vi "20-tcoupl_type_bis.vi"(3 "this":i32, 4 "type in":i32, 5 "button":i32, 6 "settings in":T1={"Auto1"=TRUE, "Auto2"=TRUE, "Rel1"=TRUE, "Rel2"=TRUE, "Filt1"=TRUE, "Filt2"=TRUE, "Rate"=enum."Slow", "Range1"=enum."10mV", "Range2"=enum."100mV", "Filt3"=TRUE, "Filt4"=TRUE, "Rel temp 1"=TRUE, "Analog1"=FALSE, "Analog2"=FALSE, "Analog temp 1"=FALSE, "Digital1"=TRUE, "Digital2"=TRUE, "Digital temp 1 "=TRUE, "Window1"=enum."0,01%", "Window2"=enum."0,01%", "Window temp 1"=enum."0,01%", "RDGS1"="010", "RDGS2"="010", "RDGS temp 1"="010", "Type_type1"=TRUE, "Type_type2"=TRUE, "Type_type temp 1"=TRUE, "LSync"=FALSE, "Unit"=enum."C", "Sens"=TRUE, "Type tcoupl"=enum."J", "Junc"=TRUE, "prevState"=0, "Rel temp 2"=TRUE, "Analog temp 2"=FALSE, "Digital temp 2"=TRUE, "Type_type temp 2"=TRUE, "RDGS temp 2"="010", "Window temp 2"=enum."0,01%", "addres"=""}) -> (0 "next state":i32, 1 "type  out":i32, 2 "settings out":T1)   [LabVIEW 2017]
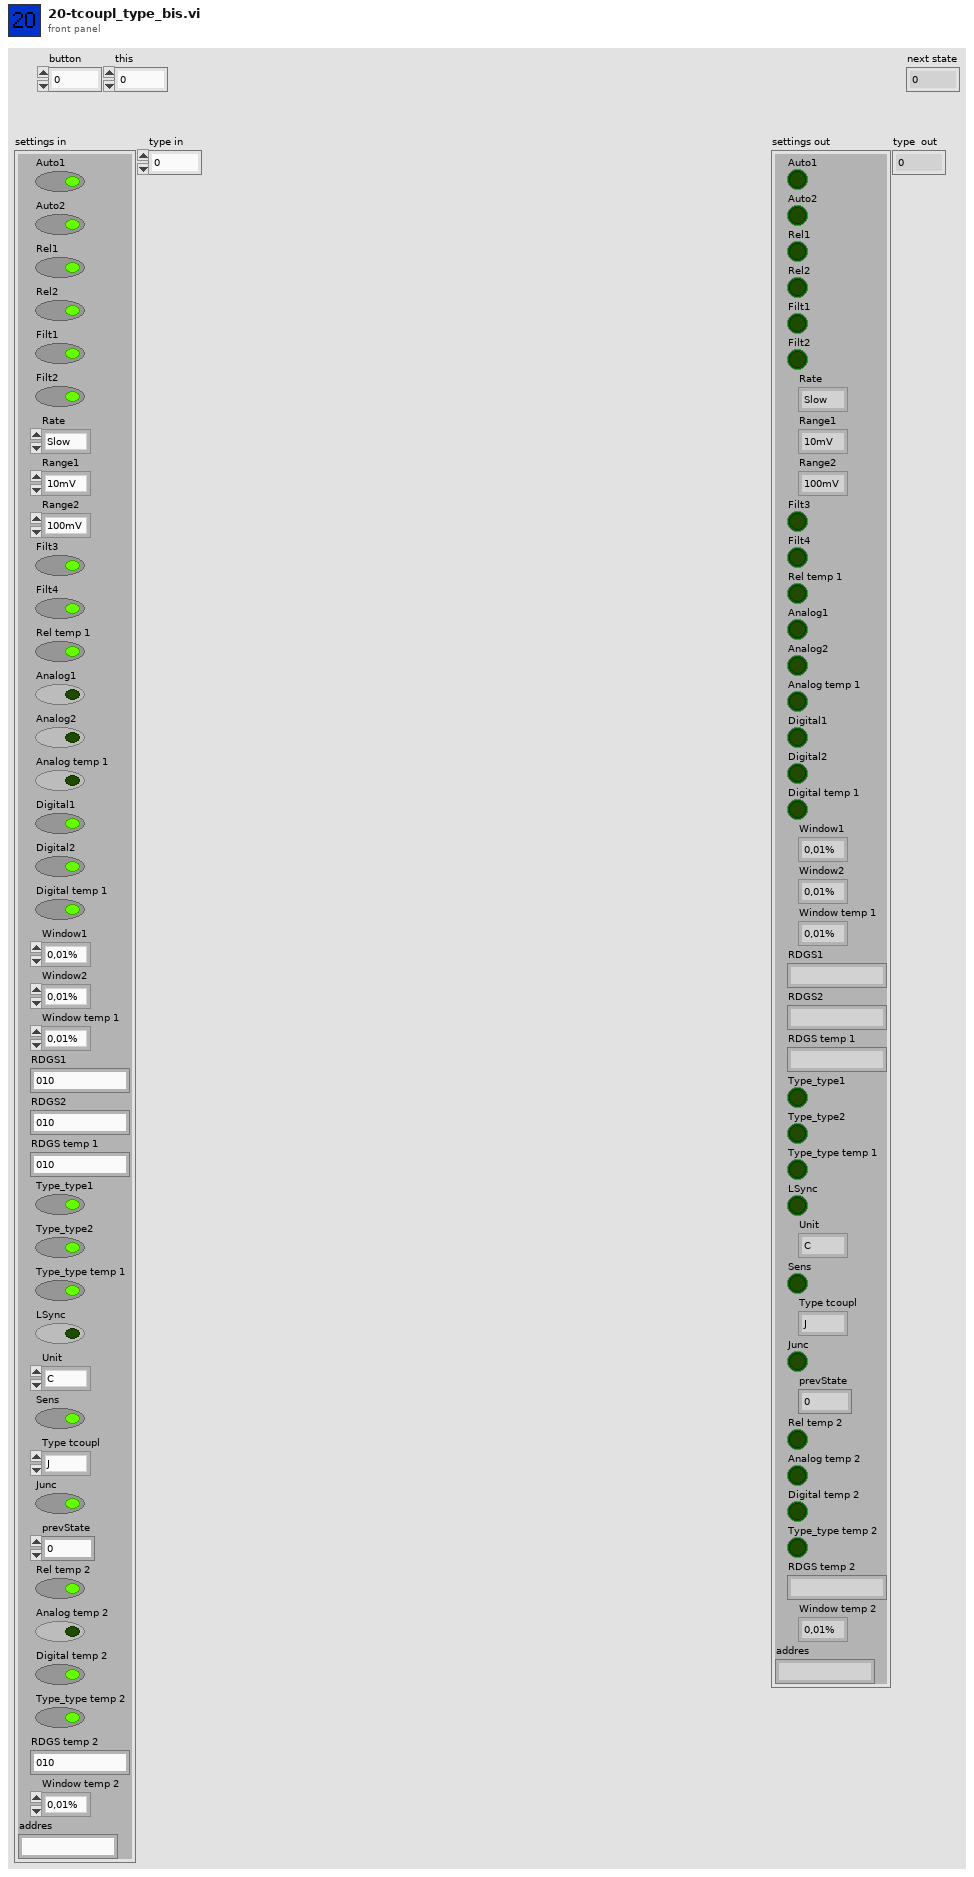
[diagram p1: front panel]
types:
  T1 = cluster{"Auto1":bool, "Auto2":bool, "Rel1":bool, "Rel2":bool, "Filt1":bool, "Filt2":bool, "Rate":enum16{"Slow", "Med", "Fast"}, "Range1":enum16{"10mV", "100mV", "1V", "10V", "100V"}, "Range2":enum16{"100mV", "1V", "10V"}, "Filt3":bool, "Filt4":bool, "Rel temp 1":bool, "Analog1":bool, "Analog2":bool, "Analog temp 1":bool, "Digital1":bool, "Digital2":bool, "Digital temp 1 ":bool, "Window1":enum16{"0,01%", "0,1%", "1%", "10%", "None"}, "Window2":enum16{"0,01%", "0,1%", "1%", "10%", "None"}, "Window temp 1":enum16{"0,01%", "0,1%", "1%", "10%", "None"}, "RDGS1":string, "RDGS2":string, "RDGS temp 1":string, "Type_type1":bool, "Type_type2":bool, "Type_type temp 1":bool, "LSync":bool, "Unit":enum16{"C", "K", "F"}, "Sens":bool, "Type tcoupl":enum16{"J", "K", "T", "E", "R", "S", "B", "N"}, "Junc":bool, "prevState":i32, "Rel temp 2":bool, "Analog temp 2":bool, "Digital temp 2":bool, "Type_type temp 2":bool, "RDGS temp 2":string, "Window temp 2":enum16{"0,01%", "0,1%", "1%", "10%", "None"}, "addres":string}
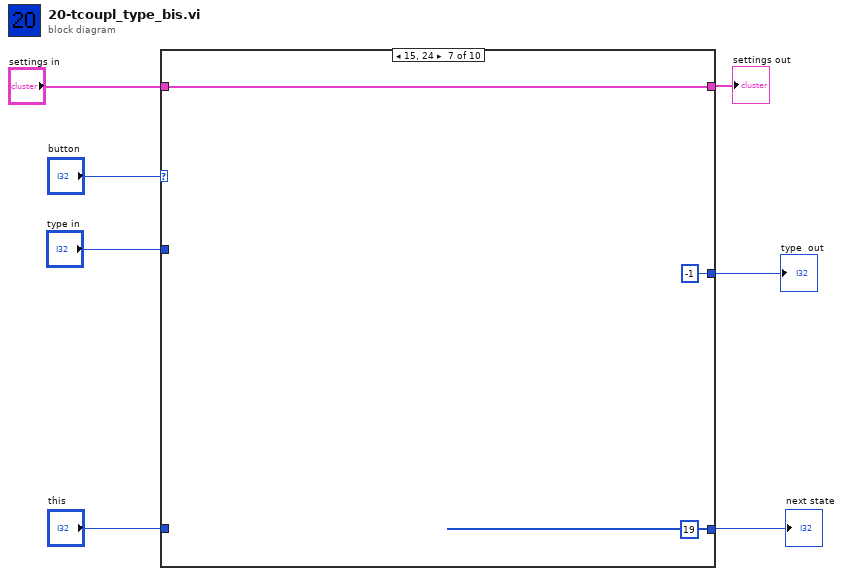
[diagram p0: block diagram]
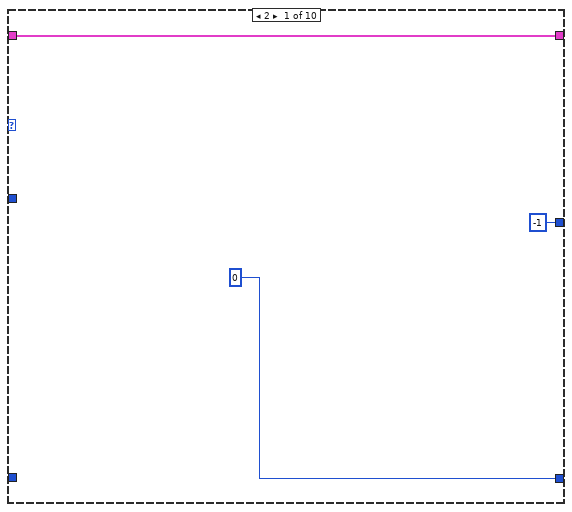
[diagram p2: hidden frame]
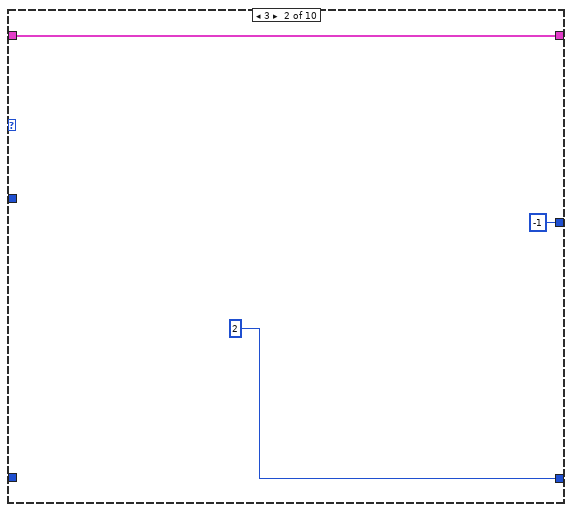
[diagram p3: hidden frame]
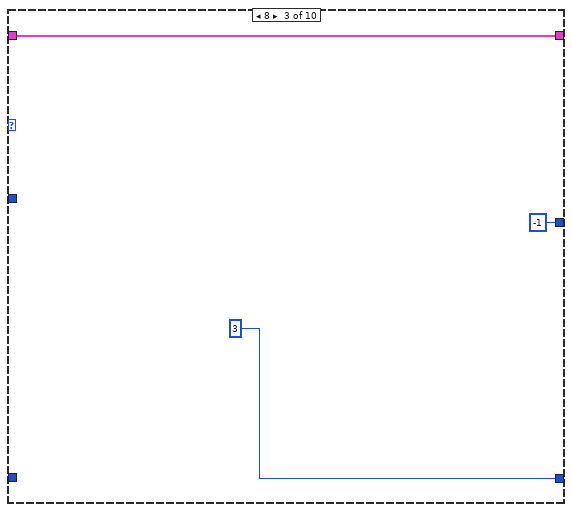
[diagram p4: hidden frame]
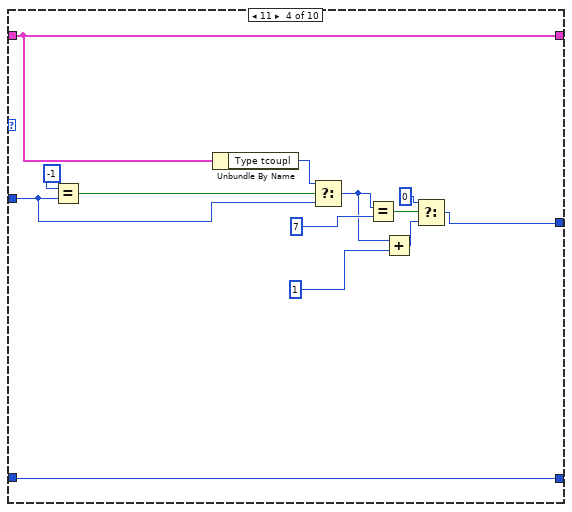
[diagram p5: hidden frame]
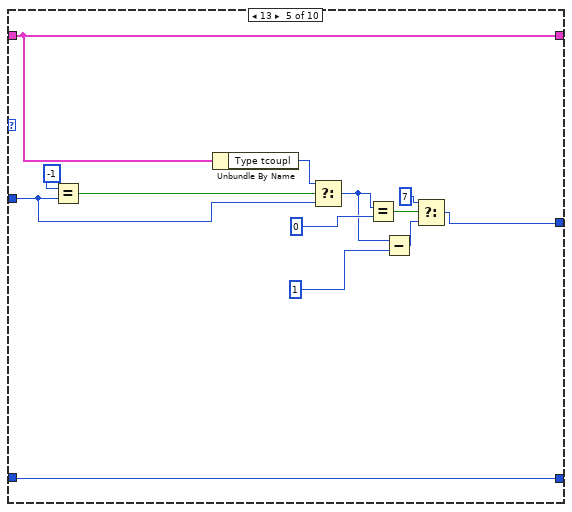
[diagram p6: hidden frame]
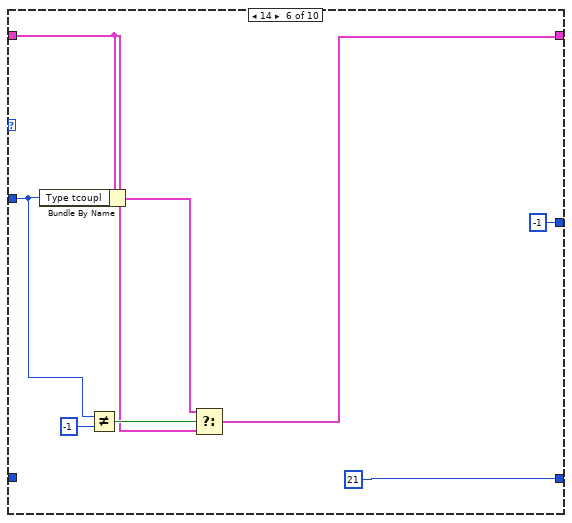
[diagram p7: hidden frame]
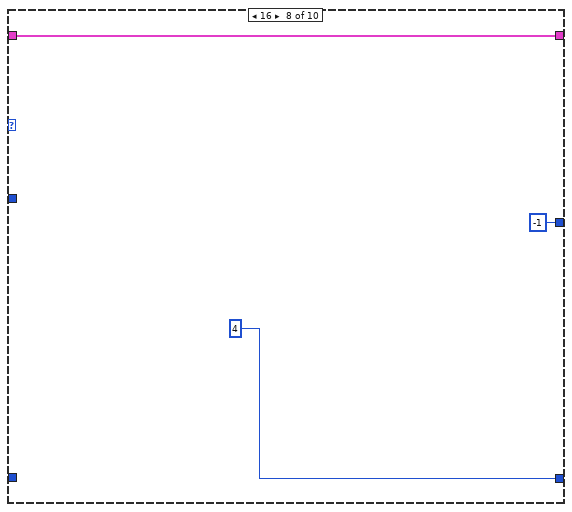
[diagram p8: hidden frame]
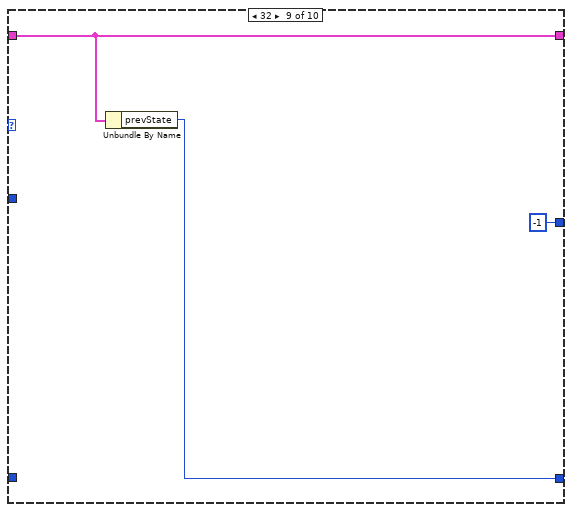
[diagram p9: hidden frame]
diagram:
  n1 = case shown="15, 24" "button" {
    tunnel: [0 ("this") 2 3 w29 w42 21 ("this") 19 ("prevState") 4 w58 w61] -> w5
    tunnel: "this" -> [_ _ _ w29 w42 _ _ _ _ w61]
    tunnel: "settings in" -> [w10 w12 w15 w26 w39 w47 w53 w55 w59 w62]
    tunnel: [w10 w12 w15 w26 w39 w44 w53 w55 w59 w62] -> w3
    tunnel: "type in" -> [_ _ _ w27 w40 w46 _ _ _ w60]
    tunnel: [-1 ("window in") -1 ("window in") -1 ("window in") w24 w37 -1 ("window in") -1 ("window in") -1 ("window in") -1 ("window in") w60] -> w1
    frame 2 {
    }
    frame 3 {
    }
    frame 8 {
    }
    frame 11 {
      n2 = Equal?(x=-1, y=w27) -> (x = y?=w28:bool)
      n3 = Unbundle By Name(w26) -> ("Type tcoupl"=w18:enum16{"J", "K", "T", "E", "R", "S", "B", "N"})
      n4 = Select(t=w18, s=w28, f=w27) -> (s? t:f=w17:i32)
      n5 = Equal?(x=w17, y=7) -> (x = y?=w22:bool)
      n6 = Add(x=w17, y=1) -> (x+y=w23:i32)
      n7 = Select(t=0, s=w22, f=w23) -> (s? t:f=w24:i32)
    }
    frame 13 {
      n8 = Equal?(x=-1, y=w40) -> (x = y?=w41:bool)
      n9 = Unbundle By Name(w39) -> ("Type tcoupl"=w31:enum16{"J", "K", "T", "E", "R", "S", "B", "N"})
      n10 = Select(t=w31, s=w41, f=w40) -> (s? t:f=w30:i32)
      n11 = Equal?(x=w30, y=0) -> (x = y?=w35:bool)
      n12 = Subtract(x=w30, y=1) -> (x-y=w36:i32)
      n13 = Select(t=7, s=w35, f=w36) -> (s? t:f=w37:i32)
    }
    frame 14 {
      n14 = Bundle By Name(cluster=w47, "Type tcoupl"=w46) -> (w45:T1)
      n15 = Not Equal?(x=w46, y=-1) -> (x != y?=w48:bool)
      n16 = Select(t=w45, s=w48, f=w47) -> (s? t:f=w44:T1)
    }
    frame 15, 24 {
    }
    frame 16 {
    }
    frame 32 {
      n17 = Unbundle By Name(w59) -> ("prevState"=w58:i32)
    }
    frame Default {
    }
  }
  "next state" <- w5
  "settings out" <- w3
  "type  out" <- w1
